vi "OUTPUT.vi"(0 "Bin_I":T3, 1 "sign":bool, 5 "flags_I":T2, 7 "C":bool, 9 "Read":bool, 11 "Reset":bool) -> (4 "Digitals":T1, 8 "Bin_O":T3, 15 "Flags_O":T2)   [LabVIEW 2017]
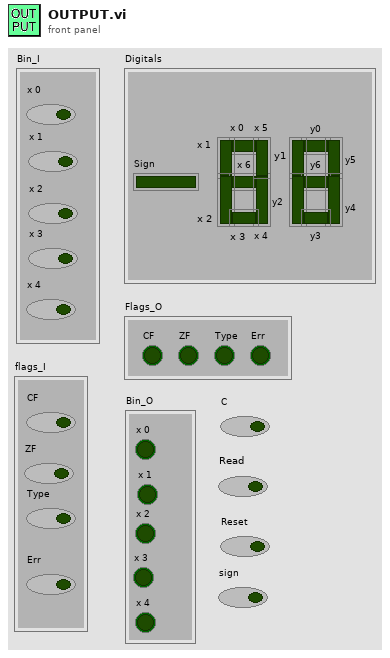
[diagram p1: front panel]
types:
  T1 = cluster{"y0":bool, "y1":bool, "y5":bool, "y6":bool, "y2":bool, "y4":bool, "y3":bool, "x 0":bool, "x 1":bool, "x 6":bool, "x 4":bool, "x 2":bool, "x 5":bool, "x 3":bool, "Sign":bool}
  T2 = cluster{"CF":bool, "ZF":bool, "Type":bool, "Err":bool}
  T3 = cluster{"x 0":bool, "x 1":bool, "x 2":bool, "x 3":bool, "x 4":bool}
  T4 = cluster{"Q 0":bool, "Q 1":bool, "Q 2":bool, "Q 3":bool}
  T5 = cluster{"y0":bool, "y1":bool, "y5":bool, "y6":bool, "y2":bool, "y4":bool, "y3":bool, bool, bool, bool, "dec2":bool, bool, "dec1":bool, bool, "sign":bool}
  T6 = cluster{"Q 0":bool, "Q 1":bool, "Q 2":bool, "Q 3":bool, "Q 4":bool}
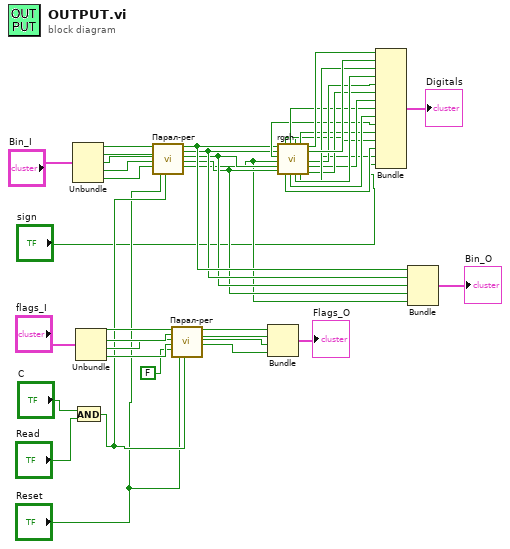
[diagram p0: block diagram]
diagram:
  n1 = Unbundle("Bin_I") -> ("x 0"=w39:bool, "x 1"=w38:bool, "x 2"=w37:bool, "x 3"=w36:bool, "x 4"=w35:bool)
  n2 = And(x="C", y="Read") -> (x .and. y?=w12:bool)
  n3 = Unbundle("flags_I") -> ("CF"=w34:bool, "ZF"=w33:bool, "Type"=w32:bool, "Err"=w31:bool)
  n4 = call "Парал-рег.vi"("d 1"=w39, "d 2"=w38, "d 3"=w37, "d 4"=w36, "d 5"=w35, "Reset"="Reset", "C"=w12) -> ("Q 0"=w10:bool, "Q 1"=w9:bool, "Q 2"=w8:bool, "Q 3"=w3:bool, "Q 4"=w2:bool)  [unwired: 8 in]
  n5 = call "Парал-рег.vi"("d 1"=w34, "d 2"=w33, "d 3"=w32, "d 4"=w31, "d 5"=FALSE, "Reset"="Reset", "C"=w12) -> ("Q 0"=w7:bool, "Q 1"=w6:bool, "Q 2"=w5:bool, "Q 3"=w4:bool)  [unwired: 8 in, 1 out]
  n6 = Bundle("Q 0"=w7, "Q 1"=w6, "Q 2"=w5, "Q 3"=w4) -> (→"Flags_O":T4)  [unwired: 1 in]
  n7 = call "rgsh.vi"("x0"=w10, "x1"=w9, "x4"=w2, "x2"=w8, "x3"=w3) -> (2:w19:bool, 6:w17:bool, "dec1"=w16:bool, 8:w21:bool, 9:w20:bool, 10:w15:bool, "y6"=w27:bool, "dec2"=w18:bool, "y5"=w26:bool, "y0"=w29:bool, "y1"=w28:bool, "y2"=w25:bool, "y3"=w23:bool, "y4"=w24:bool)  [unwired: 1 in]
  n8 = Bundle("y0"=w29, "y1"=w28, "y5"=w26, "y6"=w27, "y2"=w25, "y4"=w24, "y3"=w23, w21, w20, w19, "dec2"=w18, w17, "dec1"=w16, w15, "sign"="sign") -> (→"Digitals":T5)  [unwired: 1 in]
  n9 = Bundle("Q 0"=w10, "Q 1"=w9, "Q 2"=w8, "Q 3"=w3, "Q 4"=w2) -> (→"Bin_O":T6)  [unwired: 1 in]
